vi "generate default line.vi"(8 "error in":errorcluster, 11 "operations table":T2) -> (0 "error out":errorcluster, 2 "line":T1)   [LabVIEW 2013, in "Profibus Module editor node.lvclass"]
uses:
  Profibus Module editor node.lvclass
  table reference.ctl
  table line.ctl
  <vilib>/NI/TBM Modules/Profibus/channel/Profibus channel.lvclass
  <vilib>/NI/Tag Bus/tag/Data Type.ctl
  permissions.ctl
  <vilib>/NI/Tag Bus/tag/tag descriptor.lvclass/tag descriptor.ctl
  <vilib>/NI/Tag Bus Module Framework/channel/TBM channel.lvclass/TBM channel.ctl
  <vilib>/NI/Tag Bus/tag/write tag name.vi
  <vilib>/NI/Tag Bus/tag/write data type.vi
  <vilib>/NI/Tag Bus Module Framework/channel/Write channel classification.vi
  <vilib>/NI/Tag Bus/tag/tag descriptor.lvclass
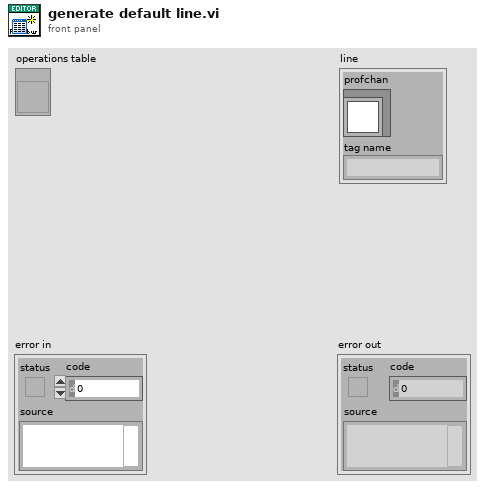
[diagram p1: front panel]
types:
  T1 = typedef "Profibus Module editor node.lvclass/table line.ctl" = cluster{"profchan":refnum<class "Profibus channel.lvclass">, "tag name":string}
  T2 = typedef "Profibus Module editor node.lvclass/table reference.ctl" = refnum<vi>
  T3 = typedef "Profibus Module editor node.lvclass/permissions.ctl" = enum32{"Read from HW", "Write to HW"}
  T4 = typedef "tag bus.lvlib/tag descriptor.lvclass/Data Type.ctl" = enum16{"Double", "Single", "I64", "I32", "I16", "I8", "U64", "U32", "U16", "U8", "Boolean", "String", "Array of Double", "Array of Single", "Array of I64", "Array of I32", "Array of I16", "Array of I8", "Array of U64", "Array of U32", "Array of U16", "Array of U8", "Array of Boolean", "Array of String"}
  T5 = typedef "TBM channel.lvclass/channel classification.ctl" = enum16{"input data", "output data", "processing parameter", "processing result"}
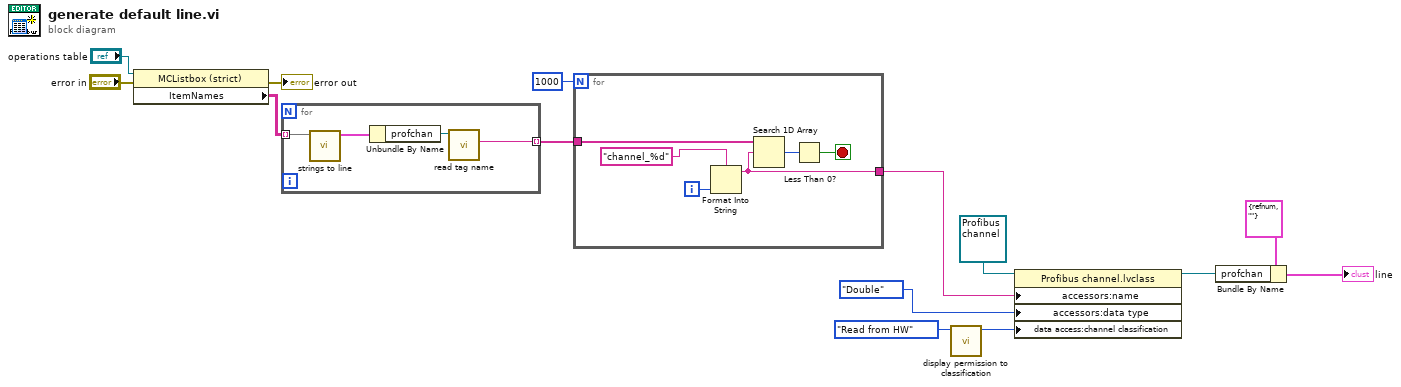
[diagram p0: block diagram]
diagram:
  n1 = property class="MCListbox (strict)"(reference="operations table", error in="error in") -> (error out=→"error out":errorcluster, "ItemNames"=w11:string[][])  [unwired: 1 out]
  n2 = for {
    tunnel: w11 -> [w18] mode=indexing
    tunnel: [w15] -> w9 mode=indexing
    n3 = call "strings to line.vi"("strings"=w18) -> ("line"=w17:T1)  [unwired: 10 in]
    n4 = Unbundle By Name(w17) -> ("profchan"=w16:refnum<class "Profibus channel.lvclass">)
    n5 = call <vilib>:"read tag name.vi"("system tag in"=w16) -> ("name"=w15:string)  [unwired: 8 in, 2 out]
  }
  n6 = for {
    N: 1000 -> [_]
    tunnel: w9 -> [w22]
    tunnel: [w19] -> w2
    i -> [w24]
    stop <- w20 stop-if-true
    n7 = Format Into String(format string="channel_%d", w24) -> (resulting string=w19:string)  [unwired: 2 in, 1 out]
    n8 = Search 1D Array(1D array=w22, element=w19) -> (index of element=w21:i32)  [unwired: 1 in]
    n9 = Less Than 0?(x=w21) -> (x < 0?=w20:bool)
  }
  n10 = call "display permission to classification.vi"("display permissions"=permissions."Read from HW") -> ("channel classification"=w1:T5)  [unwired: 10 in]
  n11 = property class="Profibus channel.lvclass"(reference=refnum<class "Profibus channel.lvclass"> refnum ("Profibus channel.lvclass"), "accessors:name"=w2, "accessors:data type"=Data_Type."Double" ("data type"), "data access:channel classification"=w1) -> (reference out=w4:refnum<class "Profibus channel.lvclass">)  [unwired: 1 in, 1 out]
  n12 = Bundle By Name(cluster=T1 {"profchan"=refnum, "tag name"=""} ("line"), "profchan"=w4) -> (→"line":T1)
